vi "4.3.vi"() -> ()   [LabVIEW 2017]
panel:
  out "输出":dbl
  in  "输入":dbl
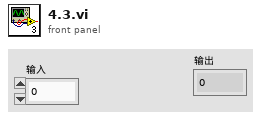
[diagram p1: front panel]
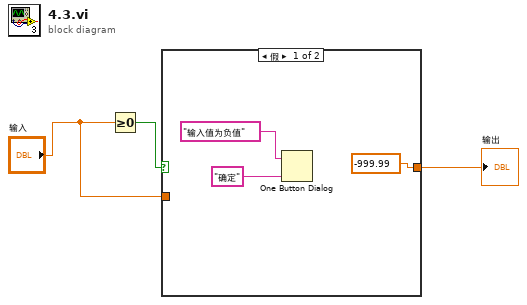
[diagram p0: block diagram]
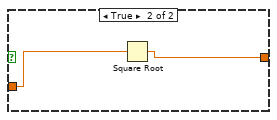
[diagram p2: hidden frame]
diagram:
  n1 = Greater Or Equal To 0?(x="输入") -> (x >= 0?=w3:bool)
  n2 = case shown="假" w3 {
    tunnel: "输入" -> [_ w8]
    tunnel: [-999.99 w7] -> w1
    frame False {
      n3 = One Button Dialog(message="输入值为负值", button name ("OK")="确定") -> ()  [unwired: 1 out]
    }
    frame True {
      n4 = Square Root(x=w8) -> (sqrt(x)=w7:dbl)
    }
  }
  "输出" <- w1
